vi "MW_Turn ON OFF.vi"(8 "错误输入（无错误）":errorcluster, 10 "start MW source?":bool, 11 "VISA引用句柄输入":refnum<visa-resource-name>) -> (0 "错误输出":errorcluster, 3 "VISA引用句柄输出":refnum<visa-resource-name>)   [LabVIEW 2016, in "Microwave Source.lvlib"]
uses:
  Microwave Source.lvlib
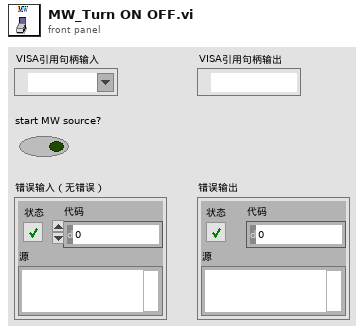
[diagram p1: front panel]
types:
  T1 = typedef "Microwave Source.lvlib/MW_ctl_DeviceType.ctl" = enum16{"R&S", "Other"}
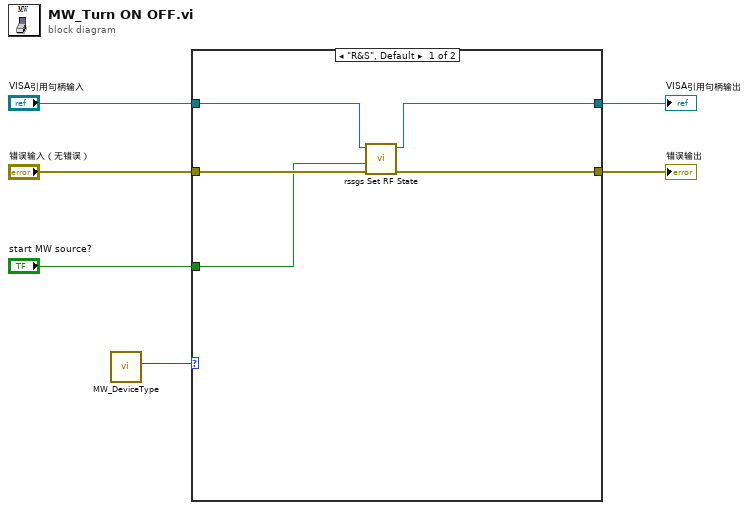
[diagram p0: block diagram]
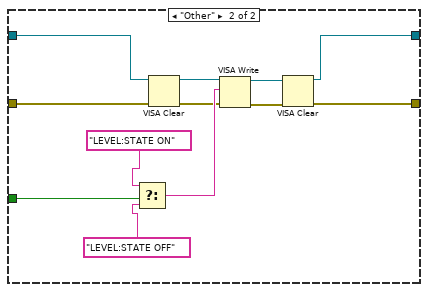
[diagram p2: hidden frame]
diagram:
  n1 = call "MW_DeviceType.vi"() -> ("DeviceType"=w1:T1)  [unwired: 11 in]
  n2 = case shown="\"R&S\", Default" w1 {
    tunnel: "start MW source?" -> [w7 w20]
    tunnel: "错误输入（无错误）" -> [w11 w17]
    tunnel: "VISA引用句柄输入" -> [w8 w16]
    tunnel: [w10 w14] -> w3
    tunnel: [w9 w12] -> w2
    frame "R&S", Default {
      n3 = call <instrlib>:"rssgs Set RF State.vi"("error in (no error)"=w11, "State (Off)"=w7, "VISA resource name"=w8) -> ("error out"=w10:errorcluster, "VISA resource name out"=w9:refnum<visa-resource-name>)  [unwired: 7 in]
    }
    frame "Other" {
      n4 = Select(t="LEVEL:STATE ON", s=w20, f="LEVEL:STATE OFF") -> (s? t:f=w23:string)
      n5 = VISA Clear(VISA resource name=w16, error in (no error)=w17) -> (VISA resource name out=w19:refnum<visa-resource-name>, error out=w18:errorcluster)
      n6 = VISA Write(VISA resource name=w19, write buffer=w23, error in (no error)=w18) -> (VISA resource name out=w13:refnum<visa-resource-name>, error out=w15:errorcluster)  [unwired: 1 out]
      n7 = VISA Clear(VISA resource name=w13, error in (no error)=w15) -> (VISA resource name out=w12:refnum<visa-resource-name>, error out=w14:errorcluster)
    }
  }
  "错误输出" <- w3
  "VISA引用句柄输出" <- w2
